vi "MultiChannelType_2D-Array-FXP.vi"(9 "error in":errorcluster, 11 "Array in":fxp<+/-,8,8>[][](array[numeric])) -> (1 "error out":errorcluster, 2 "MultiChannelType":u32, 3 "Array out":fxp<+/-,8,8>[][](array[numeric]))   [LabVIEW 2020, in "OpenLvVision_OpenCv.lvlib"]
uses:
  <vilib>/Utility/error.llb/Error Cluster From Error Code.vi
  <vilib>/ErrorRing/Error Ring.xnode
  OpenLvVision_OpenCv.lvlib
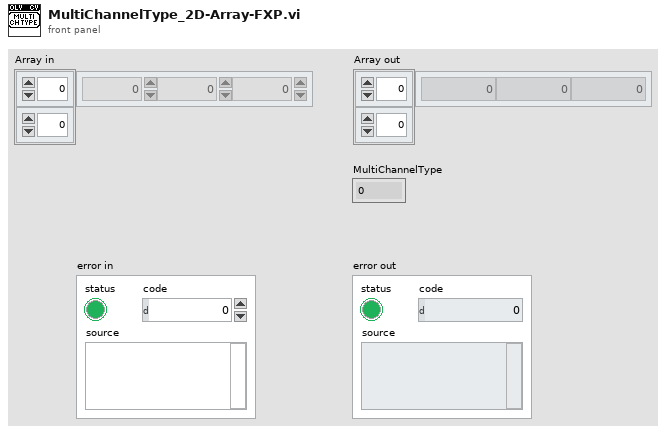
[diagram p1: front panel]
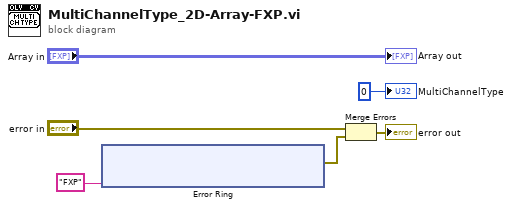
[diagram p0: block diagram]
diagram:
  n1 = xnode "Error Ring"("parameter 0"="FXP") -> ("error out"=w3:errorcluster)
  n2 = Merge Errors("error in", w3) -> (→"error out":errorcluster)
  "Array out" <- "Array in"
  "MultiChannelType" <- u32 0
